vi "Lungu Simona.vi"() -> ()   [LabVIEW 2015]
panel:
  in  "?":bool
  in  "Fisierul de salvare a datelor":path
  in  "?":bool
  in  "Selectati functia dorita":dbl(slide) scale=0.0..1.0
  in  "Valoare f":dbl
  in  "Valoare e":dbl
  in  "Valoare d":dbl
  in  "Valoare c":dbl
  in  "Valoare b":dbl
  in  "Valoare a":dbl
  out "F":dbl[](array[numeric])
  out "x2":dbl[](array[numeric])
  out "Graficul 2D al functiei f(x1,x2)":cluster{"Y":dbl[], "Y":dbl[]}[](graph)
  in  "Valoarea lui c":dbl
  in  "Valoarea lui b":dbl
  in  "Valoarea lui a":dbl
  in  "Valoarea maxima a lui x2":dbl
  in  "Valoarea minima a lui x2":dbl
  in  "Valoarea lui x1":dbl
  # "Functia polinomiala de gradul 1:"
  # "Functia polinomiala de gradul 2:"
  # "f(x1,x2)=ax1+bx2+c"
  # "f(x1,x2)=a*x1^2 + b*x1*x2 + c*x2^2 + dx1+ e*x2 +f"
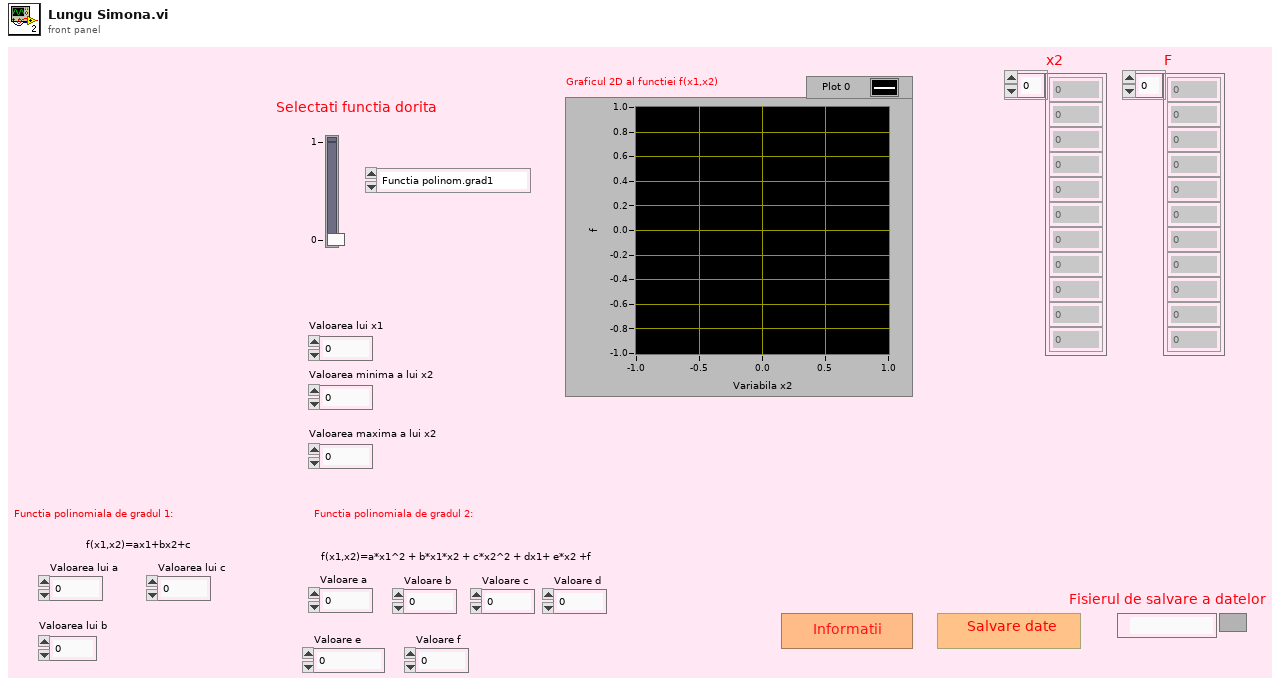
[diagram p1: front panel]
types:
  T1 = enum16{"open", "replace", "create", "open or create", "replace or create", "replace or create with confirmation"}
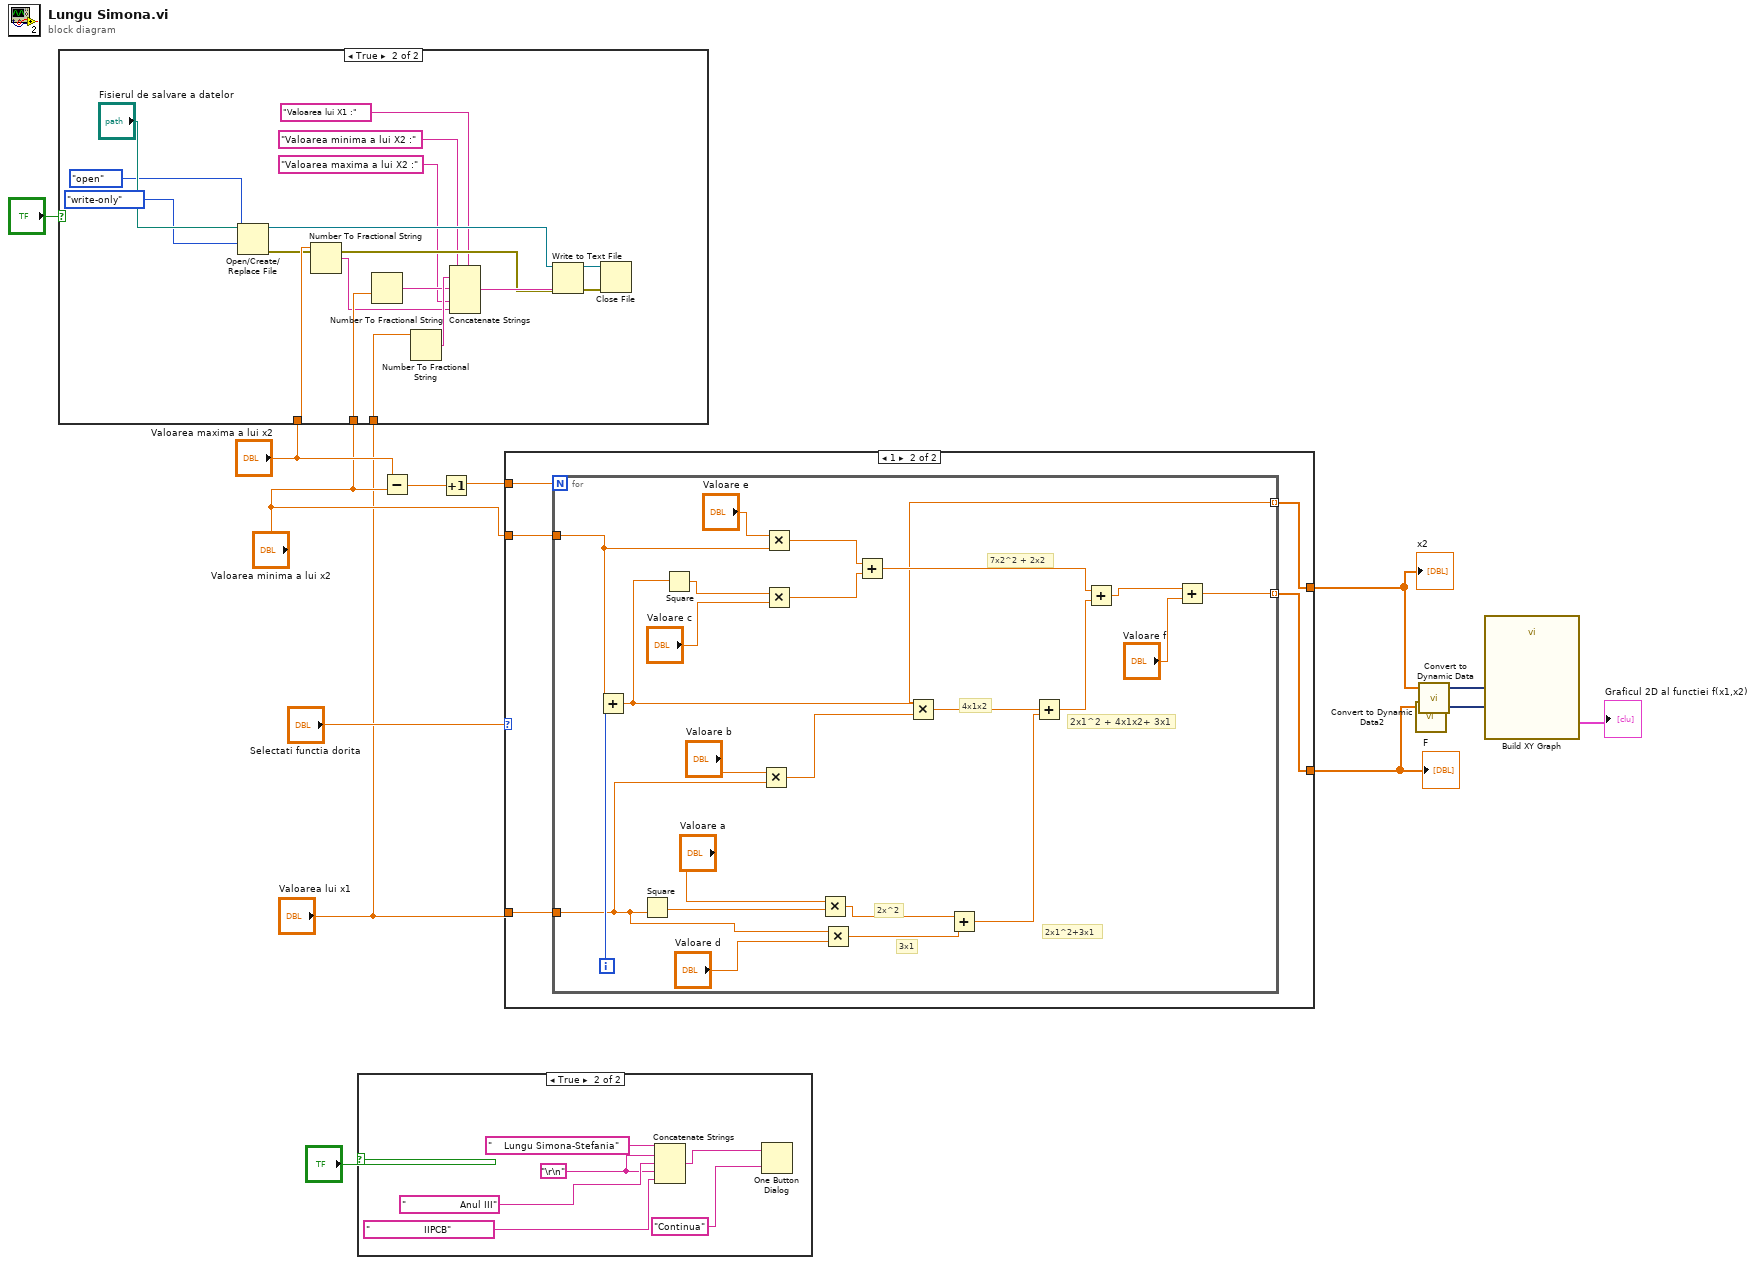
[diagram p0: block diagram]
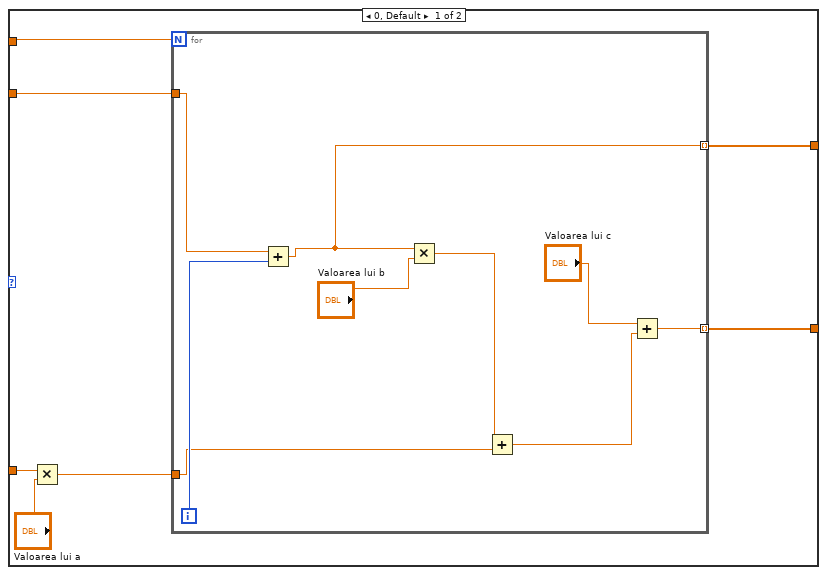
[diagram p4: hidden frame]
diagram:
  n1 = case shown="True" "?" {
    tunnel: "Valoarea maxima a lui x2" -> [_ w30]
    tunnel: "Valoarea minima a lui x2" -> [_ w29]
    tunnel: "Valoarea lui x1" -> [_ w28]
    frame False {
    }
    frame True {
      n2 = Open/Create/Replace File(file path (use dialog)="Fisierul de salvare a datelor", operation (0:open)=T1."open", access (0:read/write)=enum16{"read/write", "read-only", "write-only"}."write-only") -> (refnum out=w26:refnum<file>, error out=w25:errorcluster)  [unwired: 3 in, 1 out]
      n3 = Number To Fractional String(number=w30) -> (F-format string=w14:string)  [unwired: 3 in]
      n4 = Number To Fractional String(number=w29) -> (F-format string=w16:string)  [unwired: 3 in]
      n5 = Number To Fractional String(number=w28) -> (F-format string=w18:string)  [unwired: 3 in]
      n6 = Concatenate Strings("Valoarea lui X1 :", w18, "Valoarea minima a lui X2 :", w16, "Valoarea maxima a lui X2 :", w14) -> (w27:string)
      n7 = Write to Text File(file (use dialog)=w26, text=w27, error in=w25) -> (refnum out=w24:refnum<file>, error out=w23:errorcluster)  [unwired: 1 in, 1 out]
      n8 = Close File(refnum=w24, error in=w23) -> ()  [unwired: 2 out]
    }
  }
  n9 = case shown="True" "?" {
    frame False {
    }
    frame True {
      w34 = "\r\n"
      n10 = Concatenate Strings("    Lungu Simona-Stefania", w34, "                  Anul III", w34, "                  IIPCB") -> (w31:string)
      n11 = One Button Dialog(message=w31, button name ("OK")="Continua") -> ()  [unwired: 1 out]
    }
  }
  n12 = Subtract(x="Valoarea maxima a lui x2", y="Valoarea minima a lui x2") -> (x-y=w7:dbl)
  n13 = Increment(x=w7) -> (x+1=w6:dbl)
  n14 = case shown="1" "Selectati functia dorita" {
    tunnel: w6 -> [w43 w57]
    tunnel: "Valoarea lui x1" -> [w42 w55]
    tunnel: [w39 w53] -> w12
    tunnel: [w38 w54] -> w10
    tunnel: "Valoarea minima a lui x2" -> [w37 w56]
    frame 0, Default {
      n15 = Multiply(x=w42, y="Valoarea lui a") -> (x*y=w40:dbl)
      n16 = for {
        N: w43 -> [_]
        tunnel: w40 -> [w50]
        tunnel: [w46] -> w38 mode=indexing
        tunnel: [w45] -> w39 mode=indexing
        tunnel: w37 -> [w44]
        i -> [w52]
        n17 = Add(x=w44, y=w52) -> (x+y=w45:dbl)
        n18 = Multiply(x=w45, y="Valoarea lui b") -> (x*y=w49:dbl)
        n19 = Add(x=w49, y=w50) -> (x+y=w48:dbl)
        n20 = Add(x="Valoarea lui c", y=w48) -> (x+y=w46:dbl)
      }
    }
    frame 1 {
      n21 = for {
        N: w57 -> [_]
        tunnel: w56 -> [w71]
        tunnel: w55 -> [w73]
        tunnel: [w59] -> w54 mode=indexing
        tunnel: [w58] -> w53 mode=indexing
        i -> [w80]
        # "7x2^2 + 2x2"
        # "2x1^2 + 4x1x2+ 3x1"
        # "4x1x2"
        # "2x1^2+3x1"
        # "3x1"
        # "2x^2"
        n22 = Add(x=w71, y=w80) -> (x+y=w58:dbl)
        n23 = Square(x=w73) -> (x^2=w79:dbl)
        n24 = Square(x=w58) -> (x^2=w75:dbl)
        n25 = Multiply(x="Valoare b", y=w73) -> (x*y=w76:dbl)
        n26 = Multiply(x="Valoare e", y=w71) -> (x*y=w65:dbl)
        n27 = Multiply(x=w75, y="Valoare c") -> (x*y=w64:dbl)
        n28 = Multiply(x="Valoare a", y=w79) -> (x*y=w68:dbl)
        n29 = Multiply(x=w73, y="Valoare d") -> (x*y=w69:dbl)
        n30 = Add(x=w65, y=w64) -> (x+y=w63:dbl)
        n31 = Multiply(x=w58, y=w76) -> (x*y=w66:dbl)
        n32 = Add(x=w68, y=w69) -> (x+y=w67:dbl)
        n33 = Add(x=w66, y=w67) -> (x+y=w62:dbl)
        n34 = Add(x=w63, y=w62) -> (x+y=w61:dbl)
        n35 = Add(x=w61, y="Valoare f") -> (x+y=w59:dbl)
      }
    }
  }
  "x2" <- w12
  "F" <- w10
  n36 = call "Convert to Dynamic Data2"("Array"=w10) -> ("Dynamic Data Type"=w9:dynamicdata)  [unwired: 3 in]
  n37 = call "Convert to Dynamic Data"("Array"=w12) -> ("Dynamic Data Type"=w11:dynamicdata)  [unwired: 3 in]
  n38 = call "Build XY Graph"("Y Input"=w9, "X Input"=w11) -> ("XY Graph"=→"Graficul 2D al functiei f(x1,x2)":cluster{"X":dbl[], "Y":dbl[]}[])  [unwired: 8 in, 1 out]
